vi "BuildINSERTString.vi"(6 "values":string[](array[string]), 7 "columns":string[](array[string]), 8 "table":string) -> (3 "INSERTstring":string)   [LabVIEW 2019, in "libpqutility64.lvlib"]
uses:
  libpqutility64.lvlib
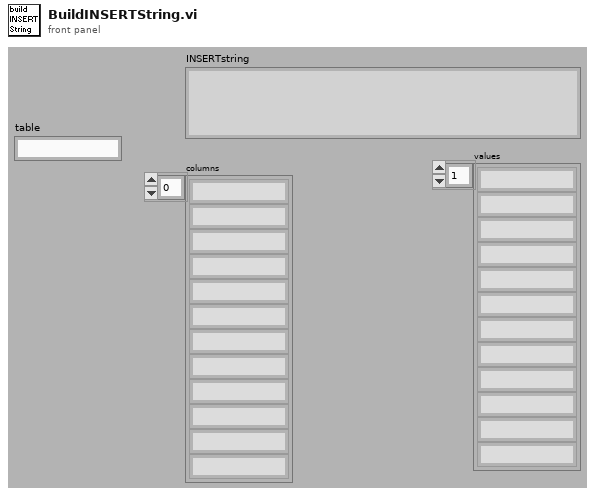
[diagram p1: front panel]
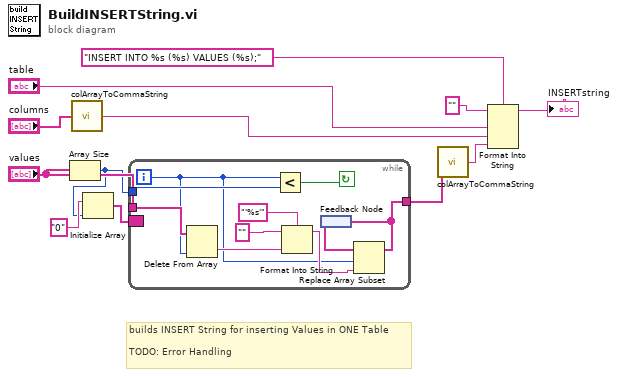
[diagram p0: block diagram]
diagram:
  # "builds INSERT String for inserting Values in ONE Table\n\nTODO: Error Handling"
  n1 = Array Size(array="values") -> (size(s)=w1:i32)
  n2 = call "colArrayToCommaString.vi"("array"="columns") -> ("comma string"=w10:string)
  n3 = Initialize Array("0" ("Element"), w1) -> (w4:string[])
  n4 = while {
    tunnel: "values" -> [w18]
    tunnel: w1 -> [w20]
    tunnel: [w14] -> w5
    border: w4 -> [_]
    i -> [w15]
    stop <- w19 continue-if-true
    n5 = Delete From Array(array=w18, index=w15) -> (deleted portion=w17:string)  [unwired: 1 in, 1 out]
    n6 = Less?(x=w15, y=w20) -> (x < y?=w19:bool)
    n7 = Format Into String(format string="'%s'" ("Format-String"), initial string="" ("Anfangsstring"), w17) -> (resulting string=w16:string)  [unwired: 1 in, 1 out]
    n8 = feedback #1() -> (w13:string[])
    n9 = Replace Array Subset(array=w13, new element=w16, index=w15) -> (w14:string[])
    n10 = feedback-in #1(w14) -> ()
  }
  n11 = call "colArrayToCommaString.vi"("array"=w5) -> ("comma string"=w11:string)
  n12 = Format Into String(format string="INSERT INTO %s (%s) VALUES (%s);" ("Format-String"), initial string="" ("Anfangsstring"), "table", w10, w11) -> (resulting string=→"INSERTstring":string)  [unwired: 1 in, 1 out]
